vi "Scan Engine Init Slot.vi"(8 "error in (no error)":errorcluster, 10 "SubPanel Ref":refnum<vi>, 11 "Node Ptr In":T1 format="%.0x") -> (0 "error out":errorcluster, 2 "RSI Module":refnum<class "RSI Module.lvclass">, 3 "Node Ptr Out":T1 format="%.0x", 5 "SubPanel Command":refnum<user-event>)   [LabVIEW 2016, in "Scan Engine Custom Device.lvlib"]
uses:
  Scan Engine Custom Device.lvlib
  Modules.lvlibp/RSI Module/SubPanel Command.ctl
  <vilib>/NI Veristand/Custom Device API/Custom Device Item Ref.ctl
  <vilib>/NI Veristand/Custom Device API/Custom Device API.lvlib
  Modules.lvlibp/RSI Module/RSI Module.lvclass
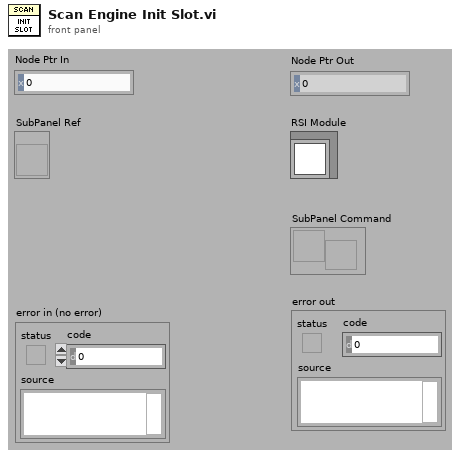
[diagram p1: front panel]
types:
  T1 = typedef "Custom Device API.lvlib/Custom Device Item Ref.ctl" = u64
  T2 = typedef "Modules.lvlibp/RSI Module.lvclass/SubPanel Command.ctl" = enum16{"Stop"}
  T3 = typedef "Modules.lvlibp/Custom Device API.lvlib/Custom Device Item Ref.ctl" = u64
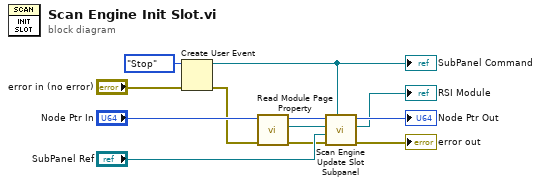
[diagram p0: block diagram]
diagram:
  n1 = Create User Event(user event datatype=SubPanel_Command."Stop" ("SubPanel Command"), error in="error in (no error)") -> (user event=w7:refnum<user-event>, error out=w4:errorcluster)
  "SubPanel Command" <- w7
  n2 = call "Read Module Page Property.vi"("error in (no error)"=w4, "Node Ptr In"="Node Ptr In") -> ("error out"=w1:errorcluster, "RSI Module"=w2:refnum<class "RSI Module.lvclass">, "Node Ptr Out"=w3:T3)  [unwired: 7 in]
  n3 = call "Scan Engine Update Slot Subpanel.vi"("SubPanel Event"=w7, "error in (no error)"=w1, "SubPanel Ref"="SubPanel Ref", "RSI Module in"=w2, "Node Ptr In"=w3) -> ("error out"=→"error out":errorcluster, "RSI Module out"=→"RSI Module":refnum<class "RSI Module.lvclass">, "Node Ptr Out"=→"Node Ptr Out":T1)  [unwired: 4 in]
